vi "Timer FGV.vi"(8 "error in (no error)":errorcluster, 11 "Mode":enum16{"Set", "Get"}(ring)) -> (0 "error out":errorcluster, 3 "Elapsed Time (sec)":string)   [LabVIEW 2015]
doc: "FGV to keep track of elapsed time in a specific test phase."
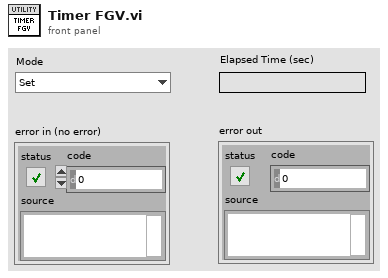
[diagram p1: front panel]
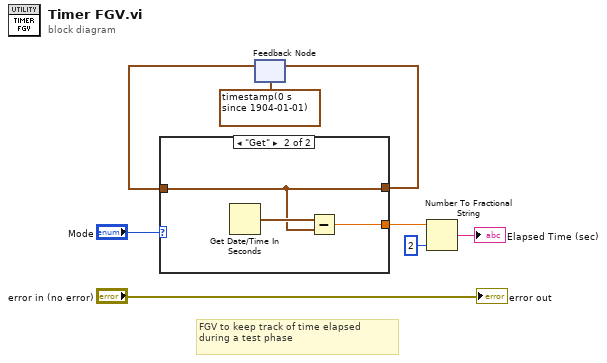
[diagram p0: block diagram]
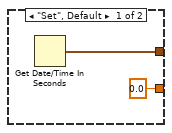
[diagram p2: hidden frame]
diagram:
  # "FGV to keep track of time elapsed\nduring a test phase"
  n1 = feedback #1(timestamp(0 s since 1904-01-01)) -> (w5:timestamp)
  n2 = case shown="\"Get\"" "Mode" {
    tunnel: w5 -> [_ w12]
    tunnel: [w10 w12] -> w4
    tunnel: [0.0 w11] -> w3
    frame "Set", Default {
      n3 = Get Date/Time In Seconds() -> (seconds since 1Jan1904=w10:timestamp)
    }
    frame "Get" {
      n4 = Get Date/Time In Seconds() -> (seconds since 1Jan1904=w13:timestamp)
      n5 = Subtract(x=w13, y=w12) -> (x-y=w11:dbl)
    }
  }
  n6 = feedback-in #1(w4) -> ()
  n7 = Number To Fractional String(number=w3, precision (6)=i16 2) -> (F-format string=→"Elapsed Time (sec)":string)  [unwired: 2 in]
  "error out" <- "error in (no error)"
